vi "PBKDF2 Derive Key (Random Salt).vi"(5 "Key length (64 bytes)":i32=64, 7 "HashingAlgorithm (SHA512)":T1=enum."SHA512", 8 "error in (no error)":errorcluster, 9 "iterations (210000)":i32=210000, 10 "saltSize (16 bytes)":i32=16, 11 "Password":string) -> (0 "error out":errorcluster, 2 "Salt":u8[](array[numeric]), 3 "Derived Key":u8[](array[numeric]))   [LabVIEW 2021, in "dotNET Crypto Key Derivation.lvlib"]
doc: "Generates a key of known length from an input password. Designed to be computationally expensive to reduce vulnerability to brute force attacks. The salt must be stored with the derived key in order to check/compare it in future.\n\nOWASP 2023 recommendation to use SHA-256 with 600,000 iterations or SHA-512 with 210,000 iterations. \n\nNIST SP 800-132 requires a salt length of 128 bits (16 bytes) minimum and key length minimum of 112 bits (14 bytes)."
uses:
  dotNET Crypto Key Derivation.lvlib
  Utility/HashingAlgorithm.ctl
  Utility/dotNET Crypto Utility.lvlib
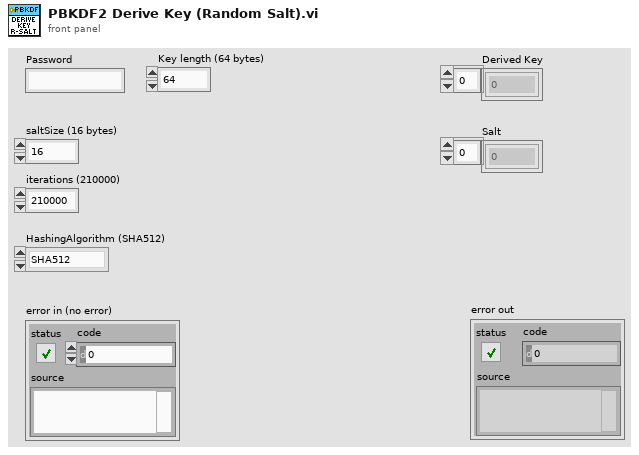
[diagram p1: front panel]
types:
  T1 = typedef "dotNET Crypto Utility.lvlib/HashingAlgorithm.ctl" = enum16{"MD5", "SHA1", "SHA256", "SHA384", "SHA512"}
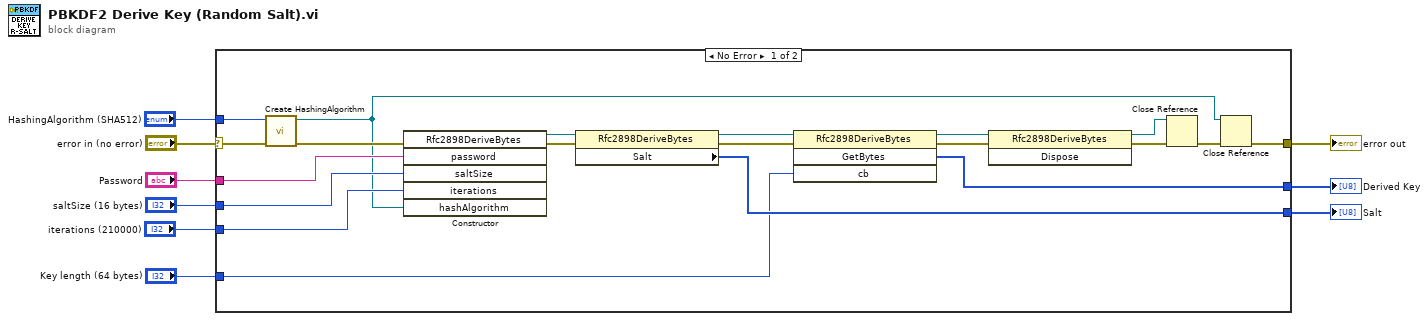
[diagram p0: block diagram]
diagram:
  n1 = case shown="No Error" "error in (no error)" {
    selector: "error in (no error)" -> [w13 w30]
    tunnel: [w29 _] -> w9
    tunnel: "HashingAlgorithm (SHA512)" -> [w28 _]
    tunnel: "saltSize (16 bytes)" -> [w27 _]
    tunnel: "iterations (210000)" -> [w26 _]
    tunnel: "Password" -> [w25 _]
    tunnel: [w24 _] -> w4
    tunnel: "Key length (64 bytes)" -> [w22 _]
    tunnel: [w11 w30] -> w2
    frame No Error {
      n2 = call "Create HashingAlgorithm.vi"("error in (no error)"=w13, "HashingAlgorithm"=w28) -> ("error out"=w14:errorcluster, "Hashing Algorithm"=w10:refnum<k24>)  [unwired: 8 in]
      n3 = constructor class="Rfc2898DeriveBytes"(error in=w14, "password"=w25, "saltSize"=w27, "iterations"=w26, "hashAlgorithm"=w10) -> (reference out=w23:refnum<k24>, error out=w19:errorcluster)  [unwired: 2 in, 5 out]
      n4 = property class="Rfc2898DeriveBytes"(reference=w23, error in=w19) -> (reference out=w21:refnum<k24>, error out=w20:errorcluster, "Salt"=w29:u8[])
      n5 = invoke class="Rfc2898DeriveBytes" method="GetBytes"(reference=w21, error in=w20, "cb"=w22) -> (reference out=w17:refnum<k24>, error out=w18:errorcluster, "GetBytes"=w24:u8[])  [unwired: 1 in, 1 out]
      n6 = invoke class="Rfc2898DeriveBytes" method="Dispose"(reference=w17, error in=w18) -> (reference out=w15:refnum<k24>, error out=w16:errorcluster)  [unwired: 1 in, 1 out]
      n7 = Close Reference(reference=w15, error in (no error)=w16) -> (error out=w12:errorcluster)
      n8 = Close Reference(reference=w10, error in (no error)=w12) -> (error out=w11:errorcluster)
    }
    frame Error {
    }
  }
  "Salt" <- w9
  "Derived Key" <- w4
  "error out" <- w2
